vi "OP600ZP_GlobalVariables.vi"() -> ()   [LabVIEW 2020]
uses:
  CheminDeBase.vi
  <vilib>/Utility/config.llb/Read Key (Double).vi
  OP600ZP_VGConf.vi
  <vilib>/Utility/config.llb/Read Key (String).vi
  OP500ZP_VGConf.vi
  <vilib>/Utility/config.llb/NI_LVConfig.lvlib
panel:
  out "error out 2":errorcluster caption="error out"
  out "error out":errorcluster
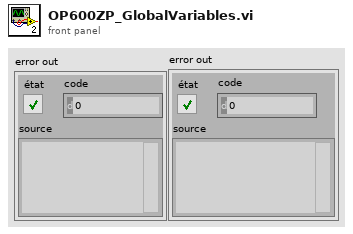
[diagram p1: front panel]
types:
  T1 = typedef "NI_LVConfig.lvlib/Config Data RefNum.ctl" = refnum<k1>
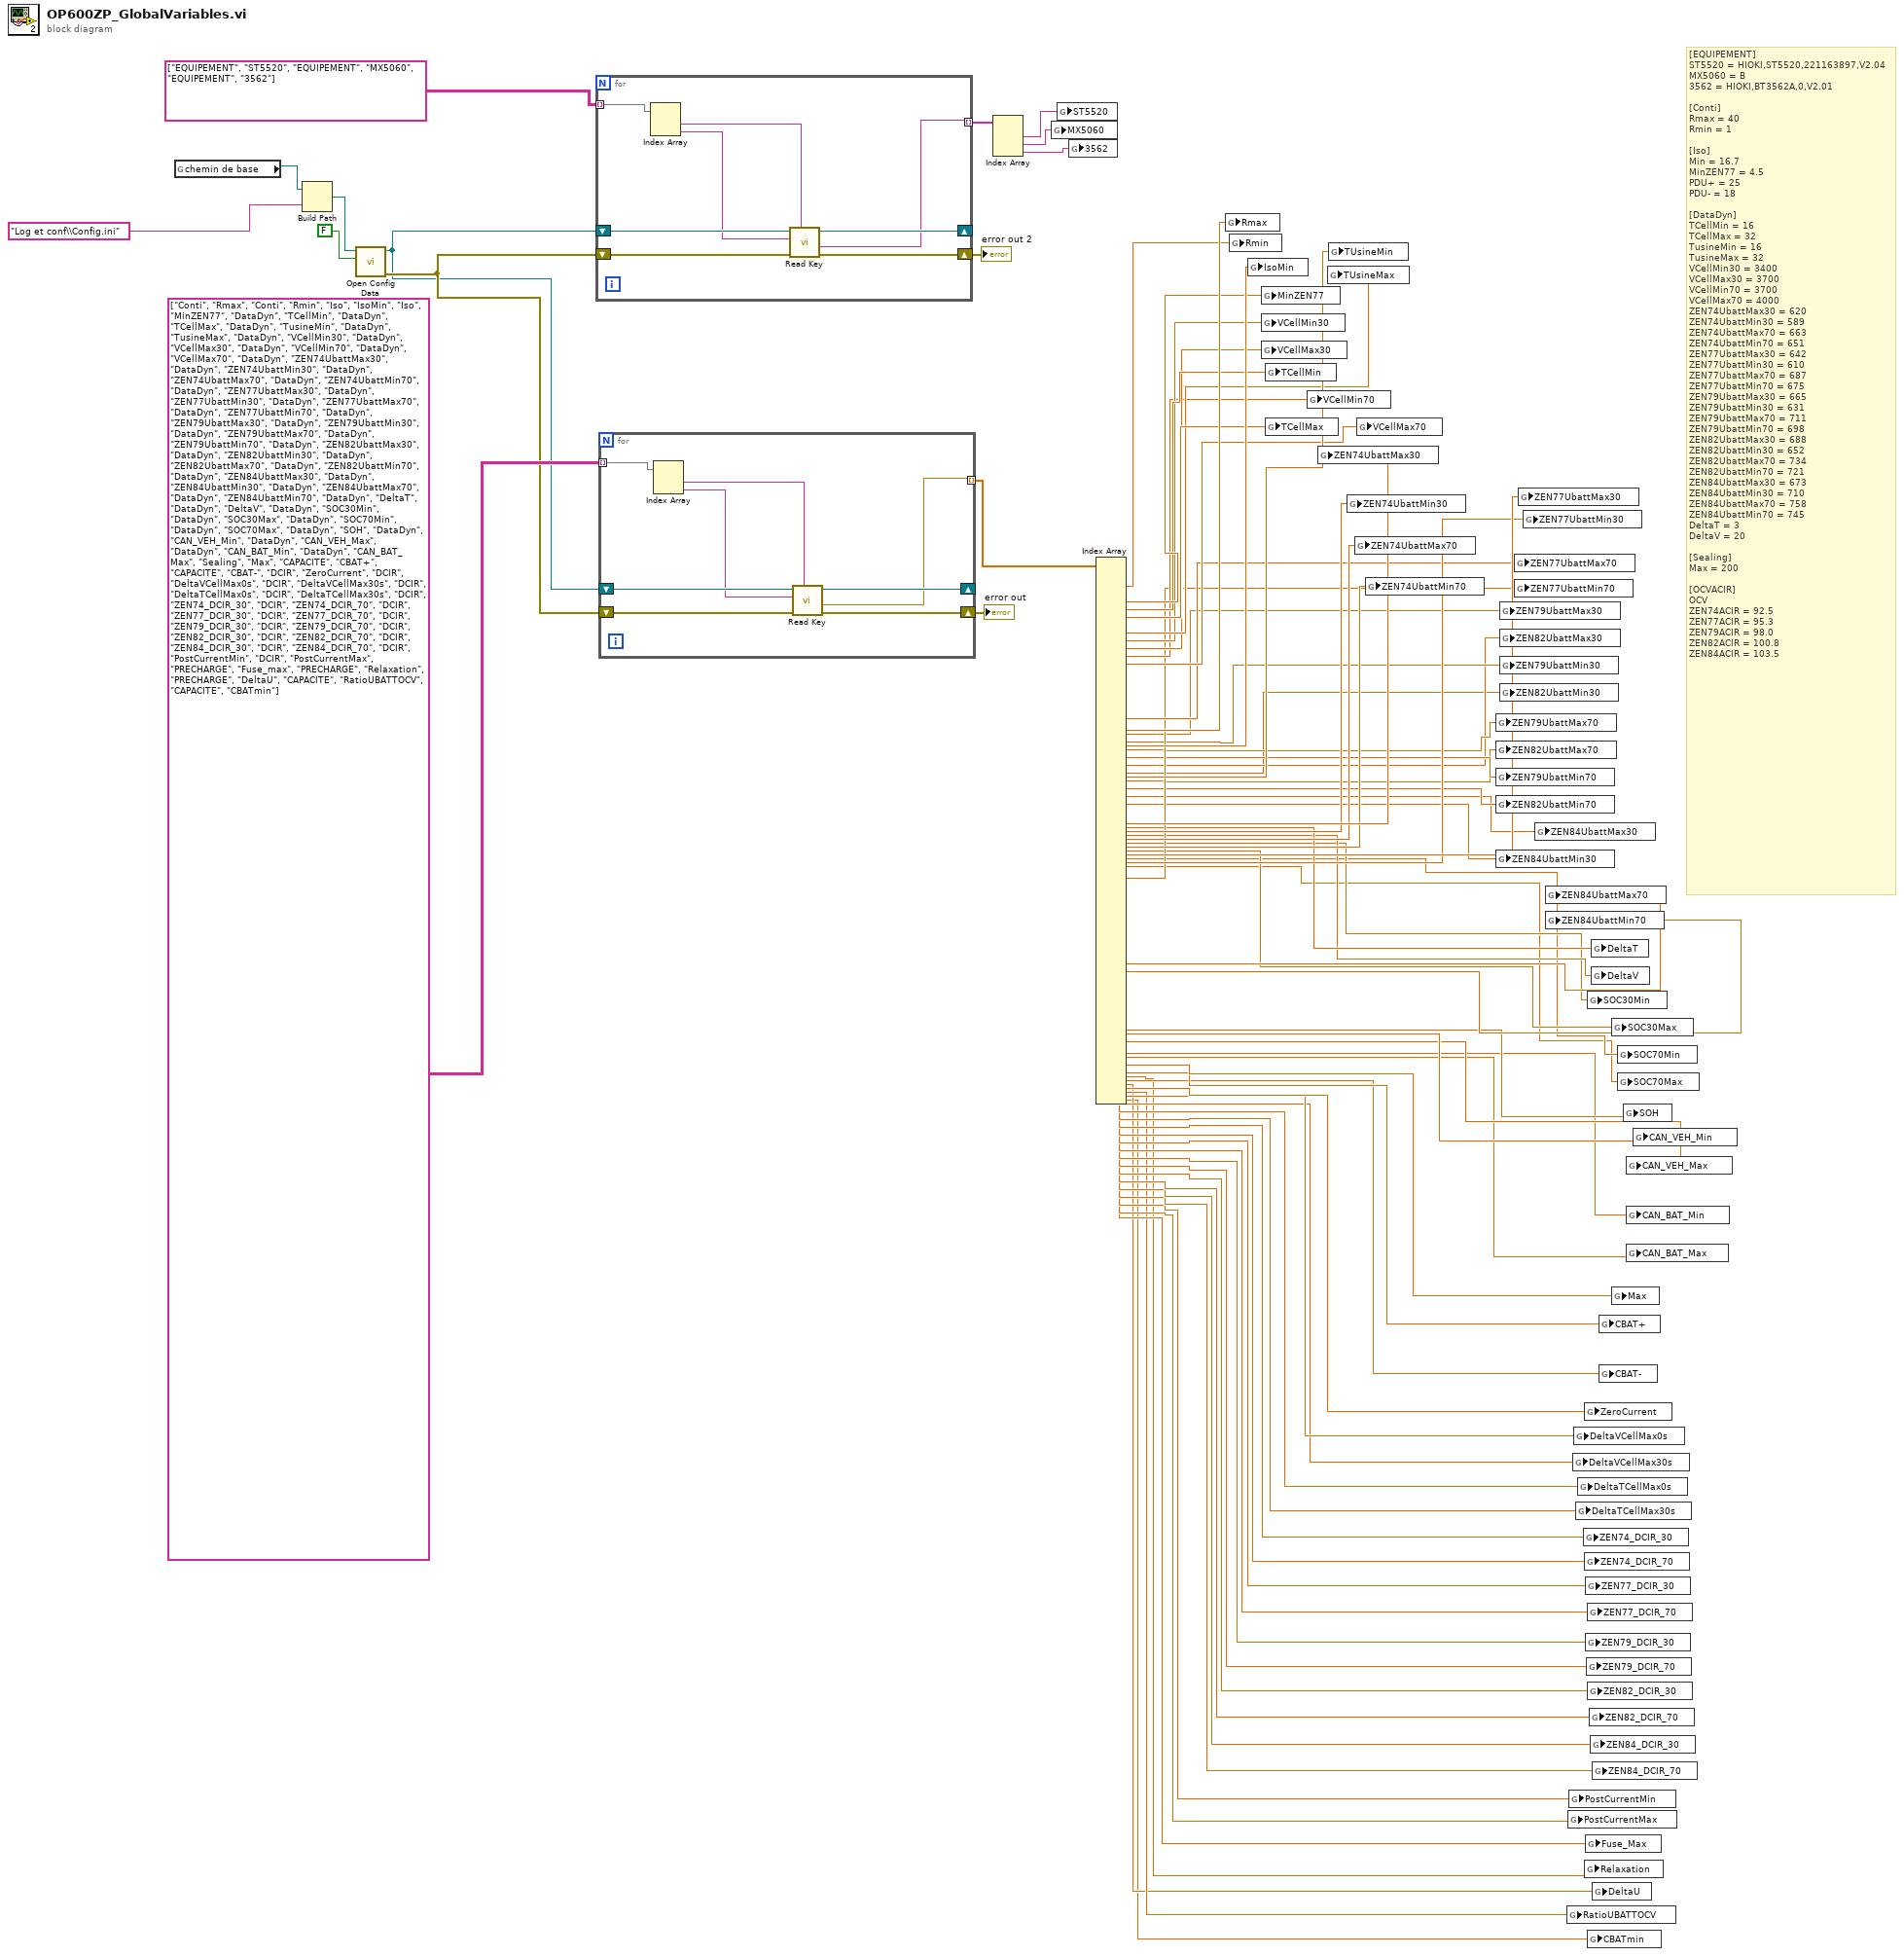
[diagram p0: block diagram]
diagram:
  # "[EQUIPEMENT]\nST5520 = HIOKI,ST5520,221163897,V2.04\t\nMX5060 = B\n3562 = HIOKI,BT3562A,0,V2.01\n\n[Conti]\nRmax = 40\nRmin = 1\n\n[Iso]\nMin = 16.7\nMinZEN77 = 4.5\nPDU+ = 25\nPDU- = 18\n\n[DataDyn]\nTCellMin = 16\nTCellMax = 32\nTusineMin = 16\nTusineMax = 32\nVCellMin30 = 3400\nVCellMax30 = 3700\nVCellMin70 = 3700\nVCellMax70 = 4000\nZEN74UbattMax30 = 620\nZEN74UbattMin30 = 589\nZEN74UbattMax70 = 663\nZEN74UbattMin70 = 651\nZEN77UbattMax30 = 642\nZEN77UbattMin30 = 610\nZEN77UbattMax70 = 687\nZEN77UbattMin70 = 675\nZEN79UbattMax30 = 665\nZEN79UbattMin30 = 631\nZEN79UbattMax70 = 711\nZEN79UbattMin70 = 698\nZEN82UbattMax30 = 688\nZEN82UbattMin30 = 652\nZEN82UbattMax70 = 734\nZEN82UbattMin70 = 721\nZEN84UbattMax30 = 673\nZEN84UbattMin30 = 710\nZEN84UbattMax70 = 758\nZEN84UbattMin70 = 745\nDeltaT = 3\nDeltaV = 20\n\n[Sealing]\nMax = 200\n\n[OCVACIR]\nOCV\nZEN74ACIR = 92.5\nZEN77ACIR = 95.3\nZEN79ACIR = 98.0\nZEN82ACIR = 100.8\nZEN84ACIR = 103.5"
  n1 = global read "CheminDeBase.vi" "chemin de base"() -> (w69:path)
  n2 = Build Path(base path=w69, name or relative path="Log et conf\\Config.ini") -> (appended path=w82:path)
  n3 = call <vilib>:"Open Config Data.vi"("create file if necessary (T)"=FALSE, "configuration file path"=w82) -> ("error out"=w73:errorcluster, "refnum"=w72:T1)  [unwired: 7 in, 1 out]
  n4 = for {
    tunnel: string[][] [["EQUIPEMENT", "ST5520"], ["EQUIPEMENT", "MX5060"], ["EQUIPEMENT", "3562"]] -> [w88] mode=indexing
    shift-right: [w89] -> w70
    shift-left: w73 -> [w91]
    shift-right: [w85] -> _
    shift-left: w72 -> [w90]
    tunnel: [w84] -> w79 mode=indexing
    n5 = Index Array(array=w88) -> (element #1=w87:string, element #2=w86:string)  [unwired: 2 in]
    n6 = call-poly <vilib>:"Read Key.vi"("section"=w87, "error in (no error)"=w91, "key"=w86, "refnum"=w90) -> ("error out"=w89:errorcluster, "value"=w84:string, "refnum out"=w85:T1)  [unwired: 4 in, 1 out]
  }
  "error out 2" <- w70
  n7 = for {
    tunnel: string[][] [["Conti", "Rmax"], ["Conti", "Rmin"], ["Iso", "IsoMin"], ["Iso", "MinZEN77"], ["DataDyn", "TCellMin"], ["DataDyn", "TCellMax"], ["DataDyn", "TusineMin"], ["DataDyn", "TusineMax"], ["DataDyn", "VCellMin30"], ["DataDyn", "VCellMax30"], ["DataDyn", "VCellMin70"], ["DataDyn", "VCellMax70"], ["DataDyn", "ZEN74UbattMax30"], ["DataDyn", "ZEN74UbattMin30"], ["DataDyn", "ZEN74UbattMax70"], ["DataDyn", "ZEN74UbattMin70"], ["DataDyn", "ZEN77UbattMax30"], ["DataDyn", "ZEN77UbattMin30"], ["DataDyn", "ZEN77UbattMax70"], ["DataDyn", "ZEN77UbattMin70"], ["DataDyn", "ZEN79UbattMax30"], ["DataDyn", "ZEN79UbattMin30"], ["DataDyn", "ZEN79UbattMax70"], ["DataDyn", "ZEN79UbattMin70"], ["DataDyn", "ZEN82UbattMax30"], ["DataDyn", "ZEN82UbattMin30"], ["DataDyn", "ZEN82UbattMax70"], ["DataDyn", "ZEN82UbattMin70"], ["DataDyn", "ZEN84UbattMax30"], ["DataDyn", "ZEN84UbattMin30"], ["DataDyn", "ZEN84UbattMax70"], ["DataDyn", "ZEN84UbattMin70"], ["DataDyn", "DeltaT"], ["DataDyn", "DeltaV"], ["DataDyn", "SOC30Min"], ["DataDyn", "SOC30Max"], ["DataDyn", "SOC70Min"], ["DataDyn", "SOC70Max"], ["DataDyn", "SOH"], ["DataDyn", "CAN_VEH_Min"], ["DataDyn", "CAN_VEH_Max"], ["DataDyn", "CAN_BAT_Min"], ["DataDyn", "CAN_BAT_Max"], ["Sealing", "Max"], ["CAPACITE", "CBAT+"], ["CAPACITE", "CBAT-"], ["DCIR", "ZeroCurrent"], ["DCIR", "DeltaVCellMax0s"], ["DCIR", "DeltaVCellMax30s"], ["DCIR", "DeltaTCellMax0s"], ["DCIR", "DeltaTCellMax30s"], ["DCIR", "ZEN74_DCIR_30"], ["DCIR", "ZEN74_DCIR_70"], ["DCIR", "ZEN77_DCIR_30"], ["DCIR", "ZEN77_DCIR_70"], ["DCIR", "ZEN79_DCIR_30"], ["DCIR", "ZEN79_DCIR_70"], ["DCIR", "ZEN82_DCIR_30"], ["DCIR", "ZEN82_DCIR_70"], ["DCIR", "ZEN84_DCIR_30"], ["DCIR", "ZEN84_DCIR_70"], ["DCIR", "PostCurrentMin"], ["DCIR", "PostCurrentMax"], ["PRECHARGE", "Fuse_max"], ["PRECHARGE", "Relaxation"], ["PRECHARGE", "DeltaU"], ["CAPACITE", "RatioUBATTOCV"], ["CAPACITE", "CBATmin"]] -> [w96] mode=indexing
    shift-right: [w97] -> w71
    shift-left: w73 -> [w99]
    shift-right: [w93] -> _
    shift-left: w72 -> [w98]
    tunnel: [w92] -> w74 mode=indexing
    n8 = Index Array(array=w96) -> (element #1=w95:string, element #2=w94:string)  [unwired: 2 in]
    n9 = call-poly <vilib>:"Read Key.vi"("section"=w95, "error in (no error)"=w99, "key"=w94, "refnum"=w98) -> ("error out"=w97:errorcluster, "value"=w92:dbl, "refnum out"=w93:T1)  [unwired: 4 in, 1 out]
  }
  "error out" <- w71
  n10 = Index Array(array=w79) -> (element #1=w78:string, element #2=w77:string, element #3=w76:string)  [unwired: 3 in]
  n11 = global write "OP500ZP_VGConf.vi" "MX5060"(w77) -> ()
  n12 = global write "OP500ZP_VGConf.vi" "ST5520"(w78) -> ()
  n13 = global write "OP500ZP_VGConf.vi" "3562"(w76) -> ()
  n14 = Index Array(array=w74) -> (element #1=w68:dbl, element #2=w7:dbl, element #3=w67:dbl, element #4=w66:dbl, element #5=w65:dbl, element #6=w64:dbl, element #7=w63:dbl, element #8=w62:dbl, element #9=w61:dbl, element #10=w60:dbl, element #11=w59:dbl, element #12=w58:dbl, element #13=w57:dbl, element #14=w56:dbl, element #15=w55:dbl, element #16=w54:dbl, element #17=w53:dbl, element #18=w52:dbl, element #19=w51:dbl, element #20=w50:dbl, element #21=w49:dbl, element #22=w48:dbl, element #23=w47:dbl, element #24=w46:dbl, element #25=w45:dbl, element #26=w44:dbl, element #27=w43:dbl, element #28=w42:dbl, element #29=w41:dbl, element #30=w40:dbl, element #31=w39:dbl, element #32=w38:dbl, element #33=w37:dbl, element #34=w36:dbl, element #35=w35:dbl, element #36=w34:dbl, element #37=w33:dbl, element #38=w32:dbl, element #39=w31:dbl, element #40=w30:dbl, element #41=w29:dbl, element #42=w28:dbl, element #43=w27:dbl, element #44=w26:dbl, element #45=w25:dbl, element #46=w24:dbl, element #47=w23:dbl, element #48=w22:dbl, element #49=w21:dbl, element #50=w20:dbl, element #51=w19:dbl, element #52=w18:dbl, element #53=w17:dbl, element #54=w16:dbl, element #55=w15:dbl, element #56=w14:dbl, element #57=w13:dbl, element #58=w12:dbl, element #59=w11:dbl, element #60=w10:dbl, element #61=w9:dbl, element #62=w8:dbl, element #63=w6:dbl, element #64=w5:dbl, element #65=w4:dbl, element #66=w2:dbl, element #67=w3:dbl, element #68=w1:dbl)  [unwired: 68 in]
  n15 = global write "OP600ZP_VGConf.vi" "Rmax"(w68) -> ()
  n16 = global write "OP600ZP_VGConf.vi" "Rmin"(w7) -> ()
  n17 = global write "OP600ZP_VGConf.vi" "IsoMin"(w67) -> ()
  n18 = global write "OP600ZP_VGConf.vi" "MinZEN77"(w66) -> ()
  n19 = global write "OP600ZP_VGConf.vi" "VCellMin30"(w61) -> ()
  n20 = global write "OP600ZP_VGConf.vi" "VCellMax30"(w60) -> ()
  n21 = global write "OP600ZP_VGConf.vi" "TCellMin"(w65) -> ()
  n22 = global write "OP600ZP_VGConf.vi" "TCellMax"(w64) -> ()
  n23 = global write "OP600ZP_VGConf.vi" "VCellMin70"(w59) -> ()
  n24 = global write "OP600ZP_VGConf.vi" "ZEN74UbattMax30"(w57) -> ()
  n25 = global write "OP600ZP_VGConf.vi" "TUsineMax"(w62) -> ()
  n26 = global write "OP600ZP_VGConf.vi" "TUsineMin"(w63) -> ()
  n27 = global write "OP600ZP_VGConf.vi" "ZEN74UbattMin30"(w56) -> ()
  n28 = global write "OP600ZP_VGConf.vi" "ZEN74UbattMax70"(w55) -> ()
  n29 = global write "OP600ZP_VGConf.vi" "VCellMax70"(w58) -> ()
  n30 = global write "OP600ZP_VGConf.vi" "ZEN74UbattMin70"(w54) -> ()
  n31 = global write "OP600ZP_VGConf.vi" "ZEN79UbattMax70"(w47) -> ()
  n32 = global write "OP600ZP_VGConf.vi" "ZEN82UbattMax70"(w43) -> ()
  n33 = global write "OP600ZP_VGConf.vi" "ZEN79UbattMin70"(w46) -> ()
  n34 = global write "OP600ZP_VGConf.vi" "ZEN82UbattMin70"(w42) -> ()
  n35 = global write "OP600ZP_VGConf.vi" "ZEN84UbattMin30"(w40) -> ()
  n36 = global write "OP600ZP_VGConf.vi" "ZEN79UbattMax30"(w49) -> ()
  n37 = global write "OP600ZP_VGConf.vi" "ZEN82UbattMax30"(w45) -> ()
  n38 = global write "OP600ZP_VGConf.vi" "ZEN79UbattMin30"(w48) -> ()
  n39 = global write "OP600ZP_VGConf.vi" "ZEN82UbattMin30"(w44) -> ()
  n40 = global write "OP600ZP_VGConf.vi" "ZEN77UbattMax70"(w51) -> ()
  n41 = global write "OP600ZP_VGConf.vi" "ZEN77UbattMin70"(w50) -> ()
  n42 = global write "OP600ZP_VGConf.vi" "ZEN77UbattMax30"(w53) -> ()
  n43 = global write "OP600ZP_VGConf.vi" "ZEN77UbattMin30"(w52) -> ()
  n44 = global write "OP600ZP_VGConf.vi" "ZEN84UbattMax30"(w41) -> ()
  n45 = global write "OP600ZP_VGConf.vi" "ZEN84UbattMax70"(w39) -> ()
  n46 = global write "OP600ZP_VGConf.vi" "ZEN84UbattMin70"(w38) -> ()
  n47 = global write "OP600ZP_VGConf.vi" "RatioUBATTOCV"(w3) -> ()
  n48 = global write "OP600ZP_VGConf.vi" "PostCurrentMax"(w6) -> ()
  n49 = global write "OP600ZP_VGConf.vi" "PostCurrentMin"(w8) -> ()
  n50 = global write "OP600ZP_VGConf.vi" "DeltaVCellMax30s"(w21) -> ()
  n51 = global write "OP600ZP_VGConf.vi" "DeltaVCellMax0s"(w22) -> ()
  n52 = global write "OP600ZP_VGConf.vi" "DeltaTCellMax30s"(w19) -> ()
  n53 = global write "OP600ZP_VGConf.vi" "DeltaTCellMax0s"(w20) -> ()
  n54 = global write "OP600ZP_VGConf.vi" "ZEN74_DCIR_30"(w18) -> ()
  n55 = global write "OP600ZP_VGConf.vi" "ZeroCurrent"(w23) -> ()
  n56 = global write "OP600ZP_VGConf.vi" "ZEN74_DCIR_70"(w17) -> ()
  n57 = global write "OP600ZP_VGConf.vi" "Relaxation"(w4) -> ()
  n58 = global write "OP600ZP_VGConf.vi" "ZEN77_DCIR_30"(w16) -> ()
  n59 = global write "OP600ZP_VGConf.vi" "ZEN79_DCIR_30"(w14) -> ()
  n60 = global write "OP600ZP_VGConf.vi" "Fuse_Max"(w5) -> ()
  n61 = global write "OP600ZP_VGConf.vi" "ZEN79_DCIR_70"(w13) -> ()
  n62 = global write "OP600ZP_VGConf.vi" "SOC30Min"(w35) -> ()
  n63 = global write "OP600ZP_VGConf.vi" "ZEN77_DCIR_70"(w15) -> ()
  n64 = global write "OP600ZP_VGConf.vi" "ZEN82_DCIR_30"(w12) -> ()
  n65 = global write "OP600ZP_VGConf.vi" "CBATmin"(w1) -> ()
  n66 = global write "OP600ZP_VGConf.vi" "ZEN82_DCIR_70"(w11) -> ()
  n67 = global write "OP600ZP_VGConf.vi" "ZEN84_DCIR_30"(w10) -> ()
  n68 = global write "OP600ZP_VGConf.vi" "DeltaT"(w37) -> ()
  n69 = global write "OP600ZP_VGConf.vi" "DeltaV"(w36) -> ()
  n70 = global write "OP600ZP_VGConf.vi" "ZEN84_DCIR_70"(w9) -> ()
  n71 = global write "OP600ZP_VGConf.vi" "DeltaU"(w2) -> ()
  n72 = global write "OP600ZP_VGConf.vi" "CBAT+"(w25) -> ()
  n73 = global write "OP600ZP_VGConf.vi" "CBAT-"(w24) -> ()
  n74 = global write "OP600ZP_VGConf.vi" "SOC30Max"(w34) -> ()
  n75 = global write "OP600ZP_VGConf.vi" "Max"(w26) -> ()
  n76 = global write "OP600ZP_VGConf.vi" "SOC70Min"(w33) -> ()
  n77 = global write "OP600ZP_VGConf.vi" "SOC70Max"(w32) -> ()
  n78 = global write "OP600ZP_VGConf.vi" "SOH"(w31) -> ()
  n79 = global write "OP600ZP_VGConf.vi" "CAN_VEH_Max"(w29) -> ()
  n80 = global write "OP600ZP_VGConf.vi" "CAN_BAT_Min"(w28) -> ()
  n81 = global write "OP600ZP_VGConf.vi" "CAN_BAT_Max"(w27) -> ()
  n82 = global write "OP600ZP_VGConf.vi" "CAN_VEH_Min"(w30) -> ()
